vi "Async Root.vi"(6 "Alias":string, 10 "Root Actors":refnum<class "Root Actors.lvclass">) -> (0 "Error out":errorcluster, 2 "Root Attributes":refnum<class "Attributes.lvclass">)   [LabVIEW 2020, in "jettl.lvlib" / "Spawn.lvlib"]
uses:
  Spawn.lvlib
  jettl.lvlib
  Attributes/Attributes.lvclass
  Base Attributes/Base Attributes.lvlib
  Transport/Transport.lvclass
  Actor/Actor.lvclass
  Msg/Msg.lvclass
  Msgs.ctl
  Attributes.ctl
  Attributes Metadata/Attributes Metadata.lvclass
  Lifetime.ctl
  Root Actors/Root Actors.lvclass
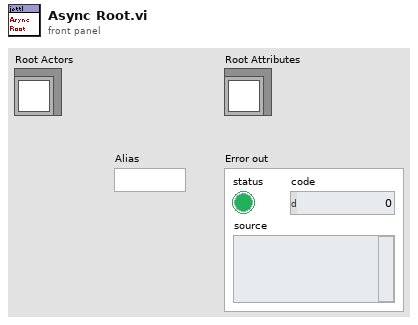
[diagram p1: front panel]
types:
  T1 = typedef "jettl.lvlib/Lifetime.ctl" = enum16{"Init", "Spawn", "Setup", "Teardown Before Running", "Running", "Stopping With Children", "Stopping Without Children", "Teardown After Running", "Stopped"}
  T2 = typedef "jettl.lvlib/Attributes.ctl" = cluster{"Attributes Metadata":refnum<class "Attributes Metadata.lvclass">, "Unified Msgs":T3, "Unified Leaf":bool, "Edge Actors":refnum<class "Actor.lvclass">[], "Core Actors":refnum<class "Actor.lvclass">[], "Parent Attributes":refnum<class "Attributes.lvclass">, "Root":bool, "Alias":string, "Transport":refnum<class "Transport.lvclass">, "VI Ref":refnum<vi>, "Actors":refnum<class "Actor.lvclass">[]}
  T3 = typedef "jettl.lvlib/Msgs.ctl" = set{refnum<class "Msg.lvclass">}
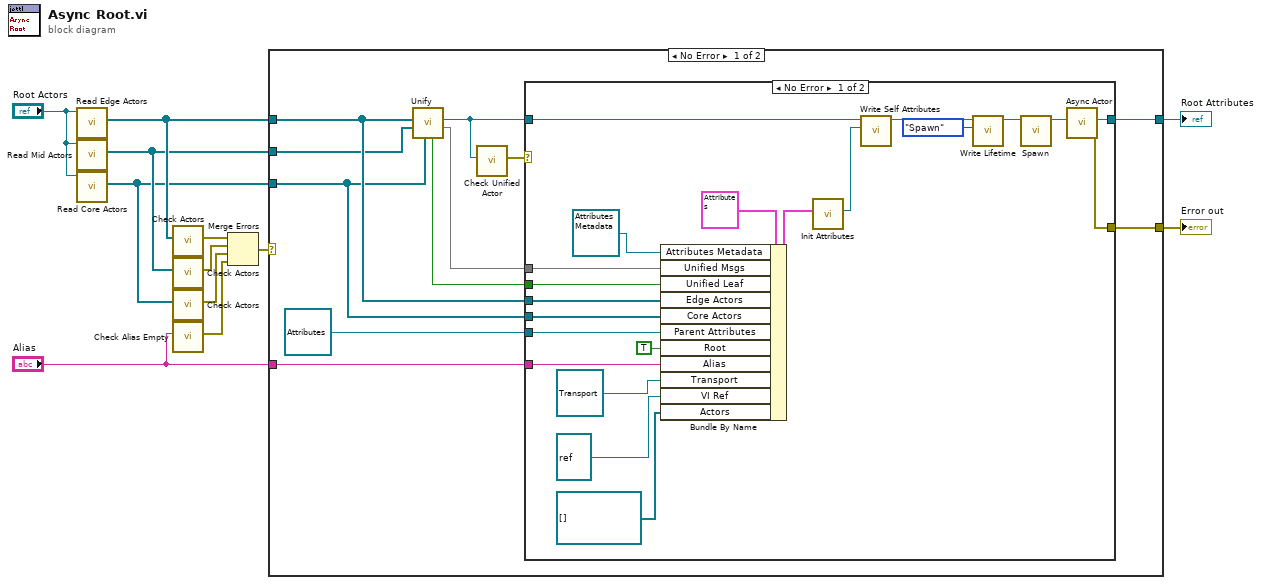
[diagram p0: block diagram]
diagram:
  n1 = call-dynamic "Read Edge Actors.vi"("Root Actors in"="Root Actors") -> ("Edge Actors"=w3:refnum<class "Actor.lvclass">[])  [unwired: 10 in]
  n2 = call-dynamic "Read Mid Actors.vi"("Root Actors in"="Root Actors") -> ("Mid Actors"=w2:refnum<class "Actor.lvclass">[])  [unwired: 10 in]
  n3 = call-dynamic "Read Core Actors.vi"("Root Actors in"="Root Actors") -> ("Core Actors"=w1:refnum<class "Actor.lvclass">[])  [unwired: 10 in]
  n4 = call "Check Actors.vi"("Actors"=w3) -> ("Error"=w5:errorcluster)  [unwired: 10 in]
  n5 = call "Check Actors.vi"("Actors"=w2) -> ("Error"=w9:errorcluster)  [unwired: 10 in]
  n6 = call "Check Actors.vi"("Actors"=w1) -> ("Error"=w6:errorcluster)  [unwired: 10 in]
  n7 = call "Check Alias Empty.vi"("Alias"="Alias") -> ("Error"=w8:errorcluster)  [unwired: 10 in]
  n8 = Merge Errors(w5, w9, w6, w8) -> (w10:errorcluster)
  n9 = case shown="No Error" w10 {
    selector: w10 -> [_ w46]
    tunnel: w3 -> [w19 _]
    tunnel: [w23 w46] -> w12
    tunnel: [w22 _] -> w11
    tunnel: "Alias" -> [w21 _]
    tunnel: w2 -> [w18 _]
    tunnel: w1 -> [w17 _]
    frame No Error {
      n10 = call "Unify.vi"("Core Actors"=w17, "Mid Actors"=w18, "Edge Actors"=w19) -> ("Unified Msgs"=w16:T3, "Unified Actor"=w15:refnum<class "Actor.lvclass">, "Unified Leaf"=w13:bool)  [unwired: 6 in]
      n11 = call "Check Unified Actor.vi"("Unified Actor"=w15) -> ("Error"=w14:errorcluster)  [unwired: 10 in]
      n12 = case shown="No Error" w14 {
        selector: w14 -> [_ w45]
        tunnel: [w44 w45] -> w23
        tunnel: [w43 _] -> w22
        tunnel: w21 -> [w41 _]
        tunnel: refnum<class "Attributes.lvclass"> refnum ("Parent Attributes") -> [w39 _]
        tunnel: w19 -> [w32 _]
        tunnel: w17 -> [w31 _]
        tunnel: w16 -> [w30 _]
        tunnel: w15 -> [w25 _]
        tunnel: w13 -> [w24 _]
        frame No Error {
          n13 = Bundle By Name(cluster=T2 {"Attributes Metadata"=refnum, "Unified Msgs"={}, "Unified Leaf"=FALSE, "Edge Actors"=[], "Core Actors"=[], "Parent Attributes"=refnum, "Root"=FALSE, "Alias"="", "Transport"=refnum, "VI Ref"=refnum, "Actors"=[]} ("Attributes"), "Attributes Metadata"=refnum<class "Attributes Metadata.lvclass"> refnum, "Unified Msgs"=w30, "Unified Leaf"=w24, "Edge Actors"=w32, "Core Actors"=w31, "Parent Attributes"=w39, "Root"=TRUE, "Alias"=w41, "Transport"=refnum<class "Transport.lvclass"> refnum, "VI Ref"=refnum<vi> refnum ("Actor Ref"), "Actors"=refnum<class "Actor.lvclass">[] []) -> (w34:T2)
          n14 = call "Init Attributes.vi"("Attributes"=w34) -> ("Attributes"=w42:refnum<class "Attributes.lvclass">)  [unwired: 10 in]
          n15 = call-dynamic "Write Self Attributes.vi"("Self Attributes"=w42, "Actor in"=w25) -> ("Actor out"=w28:refnum<class "Actor.lvclass">)  [unwired: 9 in]
          n16 = call-dynamic "Write Lifetime.vi"("Lifetime"=Lifetime."Spawn", "Actor in"=w28) -> ("Actor out"=w27:refnum<class "Actor.lvclass">)  [unwired: 9 in]
          n17 = call-dynamic "Spawn.vi"("Actor in"=w27) -> ("Actor out"=w33:refnum<class "Actor.lvclass">)  [unwired: 10 in]
          n18 = call "Async Actor.vi"("Unified Actor"=w33) -> ("Error out"=w44:errorcluster, "Attributes"=w43:refnum<class "Attributes.lvclass">)  [unwired: 9 in]
        }
        frame Error {
        }
      }
    }
    frame Error {
    }
  }
  "Error out" <- w12
  "Root Attributes" <- w11
